vi "PixelsToMeters.vi"(7 "Pict Refnum":refnum<vi>, 9 "End mouse position (px)":cluster{"X":i32, "Y":i32}, 10 "Initial mouse position (px)":cluster{"X":i32, "Y":i32}, 11 "Application reference in":refnum<vi>) -> (1 "End mouse position (m)":cluster{sgl, sgl}, 2 "Initial mouse position (m)":cluster{sgl, sgl}, 3 "Application reference out":refnum<vi>)   [LabVIEW 2021, in "Nanonis Prog Interface.lvlib"]
uses:
  Nanonis Prog Interface.lvlib
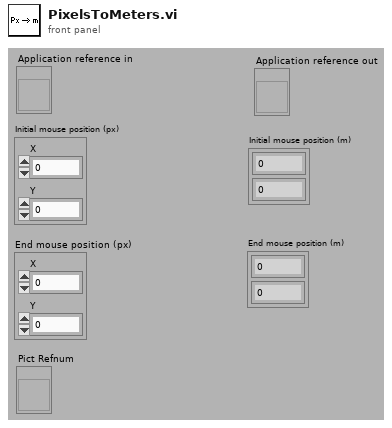
[diagram p1: front panel]
types:
  T1 = typedef "LVBoundsTypeDef.ctl" = cluster{"Width":u32, "Height":u32}
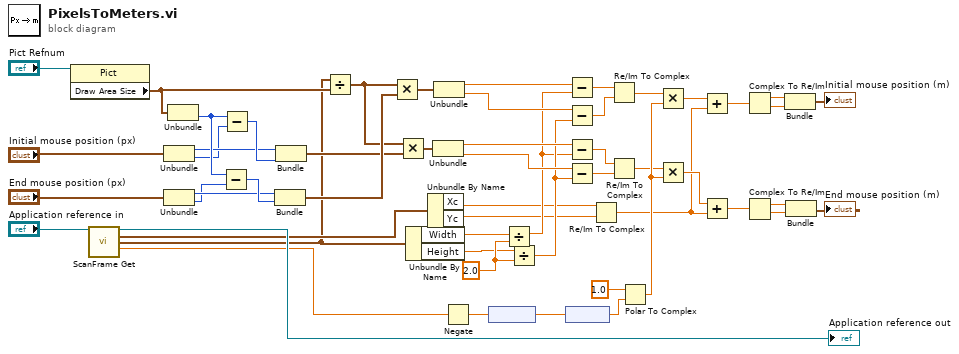
[diagram p0: block diagram]
diagram:
  w31 = sgl 2.0 ("y")
  n1 = property on="Property Node" class="Pict"(reference="Pict Refnum") -> ("Draw Area Size"=w43:T1)  [unwired: 1 in, 2 out]
  n2 = call <userlib>:"ScanFrame Get.vi"("Application ref in"="Application reference in") -> ("Application ref out"=→"Application reference out":refnum<vi>, "Center coordinates (m)"=w16:cluster{"Xc":sgl, "Yc":sgl}, "Size (m)"=w15:cluster{"Width":sgl, "Height":sgl}, "Angle (deg)"=w14:sgl)  [unwired: 10 in, 1 out]
  n3 = Unbundle("Initial mouse position (px)") -> ("X"=w46:i32, "Y"=w45:i32)
  n4 = Unbundle("End mouse position (px)") -> ("X"=w52:i32, "Y"=w50:i32)
  n5 = Unbundle(w43) -> ("Height"=w51:u32)  [unwired: 1 out]
  n6 = Subtract(x=w51, y=w50) -> (x-y=w53:u32)
  n7 = Subtract(x=w51, y=w45) -> (x-y=w47:u32)
  n8 = Bundle("X"=w52, w53) -> (w54:cluster{"X":i32, u32})  [unwired: 1 in]
  n9 = Bundle("X"=w46, w47) -> (w48:cluster{"X":i32, u32})  [unwired: 1 in]
  n10 = Divide(x=w15, y=w43) -> (x/y=w41:cluster{"Width":sgl, "Height":sgl})
  n11 = Multiply(x=w41, y=w54) -> (x*y=w39:cluster{sgl, sgl})
  n12 = Multiply(x=w41, y=w48) -> (x*y=w40:cluster{sgl, sgl})
  n13 = Unbundle By Name(w15) -> ("Width"=w34:sgl, "Height"=w30:sgl)
  n14 = Unbundle By Name(w16) -> ("Xc"=w13:sgl, "Yc"=w12:sgl)
  n15 = Unbundle(w40) -> (w37:sgl, w38:sgl)
  n16 = Unbundle(w39) -> (w35:sgl, w36:sgl)
  n17 = Negate(x=w14) -> (-x=w27:sgl)
  n18 = node(w27) -> (w25:sgl[unit])
  n19 = Divide(x=w34, y=w31) -> (x/y=w32:sgl)
  n20 = Divide(x=w30, y=w31) -> (x/y=w33:sgl)
  n21 = node(w25) -> (w26:sgl)
  n22 = Subtract(x=w35, y=w32) -> (x-y=w9:sgl)
  n23 = Subtract(x=w36, y=w33) -> (x-y=w8:sgl)
  n24 = Subtract(x=w37, y=w32) -> (x-y=w7:sgl)
  n25 = Subtract(x=w38, y=w33) -> (x-y=w6:sgl)
  n26 = Re/Im To Complex(1:w12, 2:w13) -> (0:w1:csg)
  n27 = Re/Im To Complex(1:w8, 2:w9) -> (0:w5:csg)
  n28 = Re/Im To Complex(1:w6, 2:w7) -> (0:w4:csg)
  n29 = Polar To Complex(1:w26, 2:sgl 1.0 ("r")) -> (0:w23:csg)
  n30 = Multiply(x=w5, y=w23) -> (x*y=w3:csg)
  n31 = Multiply(x=w4, y=w23) -> (x*y=w2:csg)
  n32 = Add(x=w3, y=w1) -> (x+y=w11:csg)
  n33 = Add(x=w2, y=w1) -> (x+y=w10:csg)
  n34 = Complex To Re/Im(x + iy=w11) -> (x=w22:sgl, y=w21:sgl)
  n35 = Complex To Re/Im(x + iy=w10) -> (x=w20:sgl, y=w19:sgl)
  n36 = Bundle(w22, w21) -> (→"Initial mouse position (m)":cluster{sgl, sgl})  [unwired: 1 in]
  n37 = Bundle(w20, w19) -> (→"End mouse position (m)":cluster{sgl, sgl})  [unwired: 1 in]
